vi "PROPORTIONING VALVE MicroAmp Set.vi"(4 "Refnum in":T1, 5 "milliseconds to wait":u32=100, 6 "Debug":bool, 7 "Use Micro Amp Set":bool, 8 "error in (no error)":errorcluster, 10 "Target":dbl, 11 "VISA Refnum in":refnum<visa-resource-name>) -> (0 "error out":errorcluster, 3 "VISA Refnum out":refnum<visa-resource-name>)   [LabVIEW 2016]
uses:
  MW100/Type Definitions/HEWH MW100 Channel Numbers.ctl
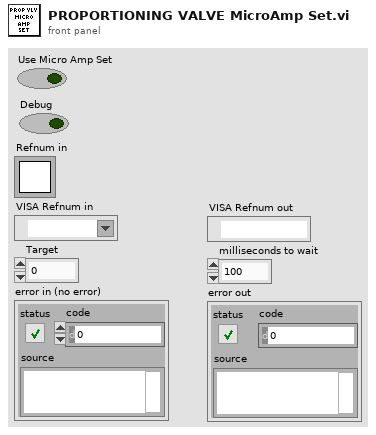
[diagram p1: front panel]
types:
  T1 = typedef "Semaphore RefNum" = refnum<k1>
  T2 = typedef "HEWH MW100 Channel Numbers.ctl" = string
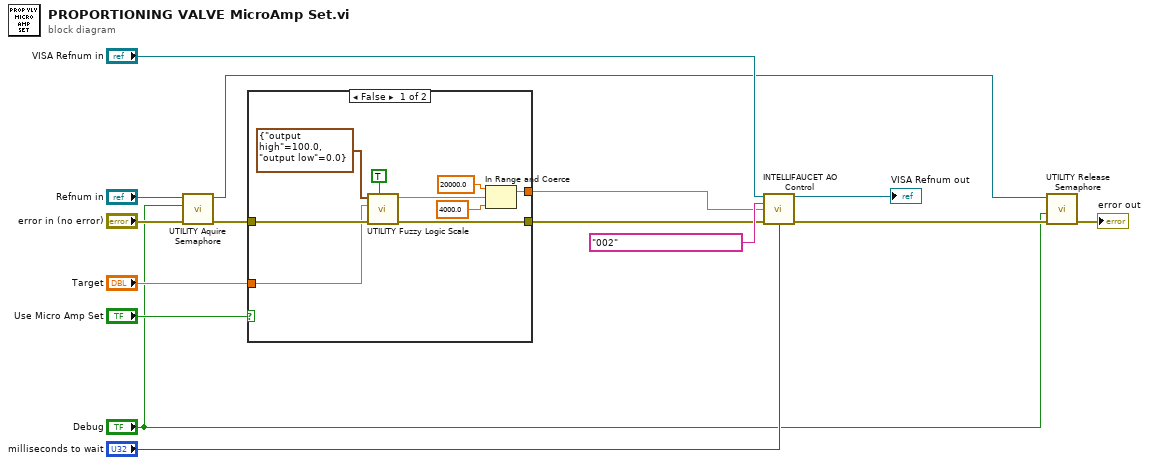
[diagram p0: block diagram]
diagram:
  n1 = call "UTILITY Aquire Semaphore.vi"("error in (no error)"="error in (no error)", "Debug"="Debug", "Refnum in"="Refnum in") -> ("error out"=w6:errorcluster, "Refnum out"=w9:T1)  [unwired: 6 in, 1 out]
  n2 = case shown="False" "Use Micro Amp Set" {
    tunnel: w6 -> [w22 w25]
    tunnel: [w21 w25] -> w5
    tunnel: [w17 w26] -> w4
    tunnel: "Target" -> [w16 w26]
    frame False {
      n3 = call "UTILITY Fuzzy Logic Scale.vi"("Convert to MicroAmp (T), Standard Output (F)"=TRUE, "Error In"=w22, "input variable"=w16, "output range"=cluster{"output high":dbl, "output low":dbl} {"output high"=100.0, "output low"=0.0}) -> ("Error Out"=w21:errorcluster, "MicroAmp"=w18:dbl)  [unwired: 6 in]
      n4 = In Range and Coerce(upper limit=20000.0, x=w18, lower limit=4000.0) -> (coerced(x)=w17:dbl)  [unwired: 1 out]
    }
    frame True {
    }
  }
  n5 = call "INTELLIFAUCET AO Control.vi"("VISA session"="VISA Refnum in", "HEWH MW100 Channel Numbers"=T2 "002", "Output Value (0)"=w4, "Error In"=w5, "milliseconds to wait"="milliseconds to wait") -> ("dup VISA session"=→"VISA Refnum out":refnum<visa-resource-name>, "error out"=w13:errorcluster)  [unwired: 9 in]
  n6 = call "UTILITY Release Semaphore.vi"("error in (no error)"=w13, "Debug"="Debug", "Refnum in"=w9) -> ("error out"=→"error out":errorcluster)  [unwired: 8 in]
